vi "显示转换.vi"(7 "显示控件":refnum<vi>, 11 "数组输入":T1(array[cluster])) -> ()   [LabVIEW 2016, in "斯坦道多参数.lvlib"]
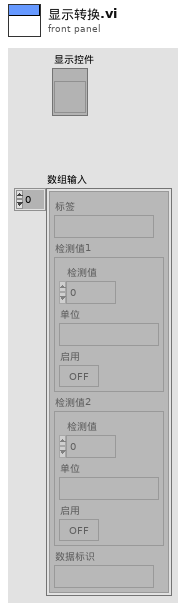
[diagram p1: front panel]
types:
  T1 = cluster{"标签":string, "检测值1":cluster{"检测值":dbl, "单位":string, "启用":bool}, "检测值2":cluster{"检测值":dbl, "单位":string, "启用":bool}, "数据标识":string}[]
  T2 = typedef "斯坦道多参数.lvlib/显示控件.ctl" = cluster{"标题背景颜色":u32, "监测值背景颜色":u32, "监测参数":string, "状态1":string, "状态2":string, "数据标识":string}
  T3 = cluster{"标签":string, "检测值1":cluster{"检测值":dbl, "单位":string, "启用":bool}, "检测值2":cluster{"检测值":dbl, "单位":string, "启用":bool}, "数据标识":string}
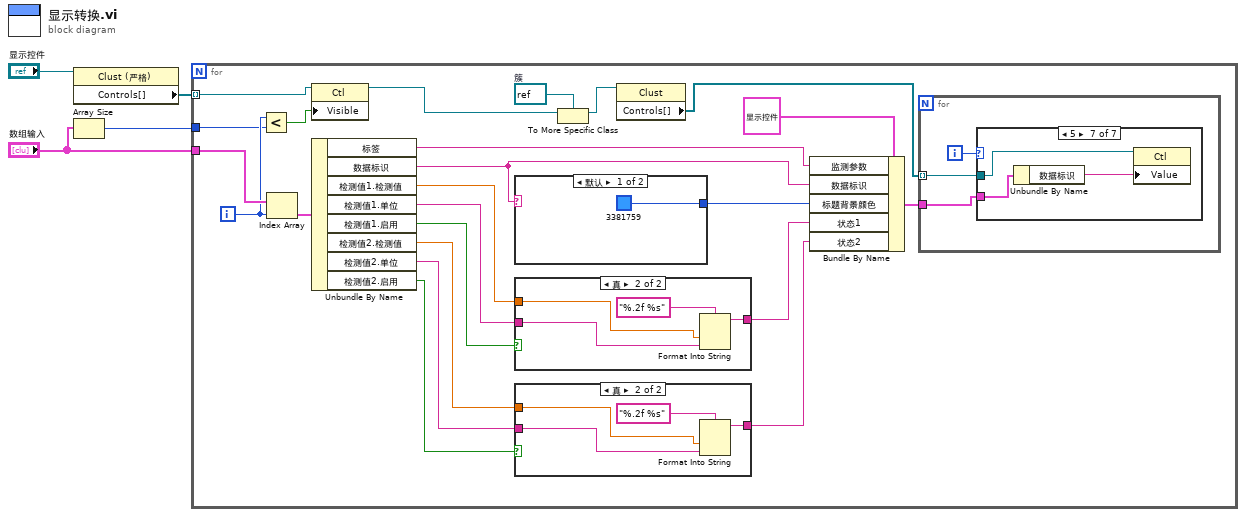
[diagram p0: block diagram]
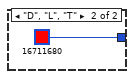
[diagram p4: hidden frame]
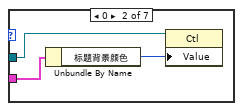
[diagram p6: hidden frame]
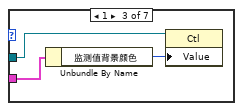
[diagram p7: hidden frame]
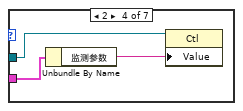
[diagram p8: hidden frame]
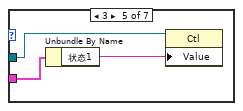
[diagram p9: hidden frame]
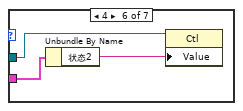
[diagram p10: hidden frame]
diagram:
  n1 = property class="Clust (严格)"(reference="显示控件") -> ("Controls[]"=w3:refnum<vi>[])  [unwired: 1 in, 2 out]
  n2 = Array Size(array="数组输入") -> (size(s)=w1:i32)
  n3 = for {
    tunnel: "数组输入" -> [w18]
    tunnel: w3 -> [w20] mode=indexing
    tunnel: w1 -> [w16]
    i -> [w17]
    w27 = refnum<vi> refnum  # 簇
    n4 = Less?(x=w17, y=w16) -> (x < y?=w15:bool)
    n5 = Index Array(array=w18, index=w17) -> (element=w19:T3)
    n6 = property class="Ctl"(reference=w20, "Visible"=w15) -> (reference out=w21:refnum<vi>)  [unwired: 1 in, 1 out]
    n7 = Unbundle By Name(w19) -> ("标签"=w22:string, "数据标识"=w13:string, "检测值1.检测值"=w12:dbl, "检测值1.单位"=w11:string, "检测值1.启用"=w10:bool, "检测值2.检测值"=w8:dbl, "检测值2.单位"=w7:string, "检测值2.启用"=w6:bool)
    n8 = case shown="默认" w13 {
      tunnel: [u32 3381759 u32 16711680] -> w14
      frame Default {
      }
      frame "D", "L", "T" {
      }
    }
    n9 = case shown="真" w10 {
      tunnel: w12 -> [_ w34]
      tunnel: w11 -> [_ w33]
      tunnel: [_ w32] -> w9
      frame False {
      }
      frame True {
        n10 = Format Into String(format string="%.2f %s" ("格式字符串"), w34, w33) -> (resulting string=w32:string)  [unwired: 2 in, 1 out]
      }
    }
    n11 = case shown="真" w6 {
      tunnel: w8 -> [_ w30]
      tunnel: w7 -> [_ w29]
      tunnel: [_ w28] -> w5
      frame False {
      }
      frame True {
        n12 = Format Into String(format string="%.2f %s" ("格式字符串"), w30, w29) -> (resulting string=w28:string)  [unwired: 2 in, 1 out]
      }
    }
    n13 = To More Specific Class(target class=w27, reference=w21) -> (specific class reference=w26:refnum<vi>)  [unwired: 1 in, 1 out]
    n14 = property class="Clust"(reference=w26) -> ("Controls[]"=w25:refnum<vi>[])  [unwired: 1 in, 2 out]
    n15 = Bundle By Name(cluster=T2 {"标题背景颜色"=3381759, "监测值背景颜色"=16777226, "监测参数"="", "状态1"="", "状态2"="", "数据标识"=""} ("显示控件"), "监测参数"=w22, "数据标识"=w13, "标题背景颜色"=w14, "状态1"=w9, "状态2"=w5) -> (w23:T2)
    n16 = for {
      tunnel: w25 -> [w40] mode=indexing
      tunnel: w23 -> [w38]
      i -> [w39]
      n17 = case shown="5" w39 {
        tunnel: w40 -> [_ w43 w46 w49 w52 w55 w58]
        tunnel: w38 -> [_ w42 w45 w48 w51 w54 w57]
        frame Default {
        }
        frame 0 {
          n18 = Unbundle By Name(w42) -> ("标题背景颜色"=w41:u32)
          n19 = property class="Ctl"(reference=w43, "Value"=w41) -> ()  [unwired: 1 in, 2 out]
        }
        frame 1 {
          n20 = Unbundle By Name(w45) -> ("监测值背景颜色"=w44:u32)
          n21 = property class="Ctl"(reference=w46, "Value"=w44) -> ()  [unwired: 1 in, 2 out]
        }
        frame 2 {
          n22 = Unbundle By Name(w48) -> ("监测参数"=w47:string)
          n23 = property class="Ctl"(reference=w49, "Value"=w47) -> ()  [unwired: 1 in, 2 out]
        }
        frame 3 {
          n24 = Unbundle By Name(w51) -> ("状态1"=w50:string)
          n25 = property class="Ctl"(reference=w52, "Value"=w50) -> ()  [unwired: 1 in, 2 out]
        }
        frame 4 {
          n26 = Unbundle By Name(w54) -> ("状态2"=w53:string)
          n27 = property class="Ctl"(reference=w55, "Value"=w53) -> ()  [unwired: 1 in, 2 out]
        }
        frame 5 {
          n28 = Unbundle By Name(w57) -> ("数据标识"=w56:string)
          n29 = property class="Ctl"(reference=w58, "Value"=w56) -> ()  [unwired: 1 in, 2 out]
        }
      }
    }
  }
